vi "example.vi"() -> ()   [LabVIEW 2015]
doc: "Created by Artem Shevelev\nshevelev.pro\nartem@shevelev.pro\nLabVIEW Portal: https://labviewportal.org/memberlist.php?mode=viewprofile&u=2340"
uses:
  cluster_example_3.ctl
  cluster_example_1.ctl
  cluster_example_2.ctl
  ini_work_Library.lvlib
panel:
  out "data2":T1
  out "data1":T1
  out "default_values":bool
  out "error out":errorcluster
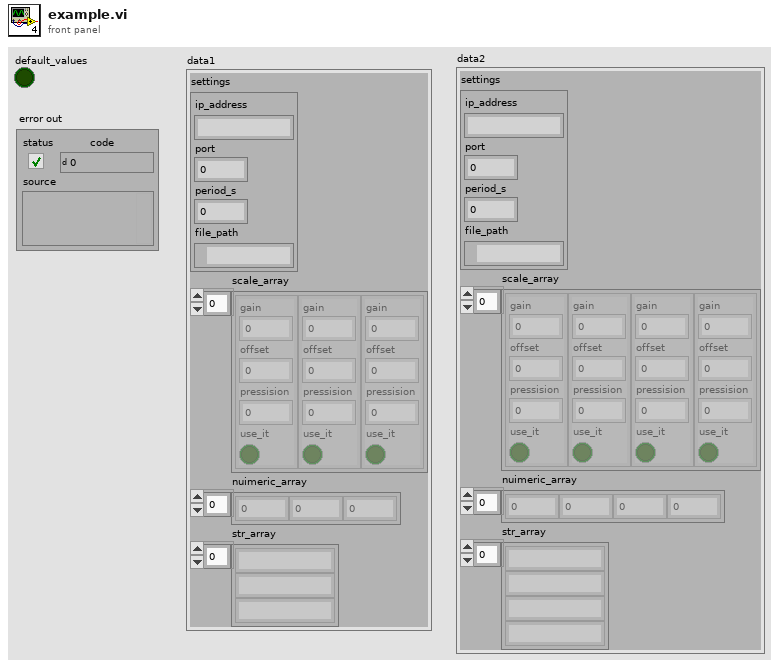
[diagram p1: front panel]
types:
  T1 = typedef "cluster_example_3.ctl" = cluster{"settings":T2, "scale_array":T3[], "nuimeric_array":dbl[], "str_array":string[]}
  T2 = typedef "cluster_example_1.ctl" = cluster{"ip_address":string, "port":i32, "period_s":dbl, "file_path":path}
  T3 = typedef "cluster_example_2.ctl" = cluster{"gain":dbl, "offset":dbl, "pressision":i32, "use_it":bool}
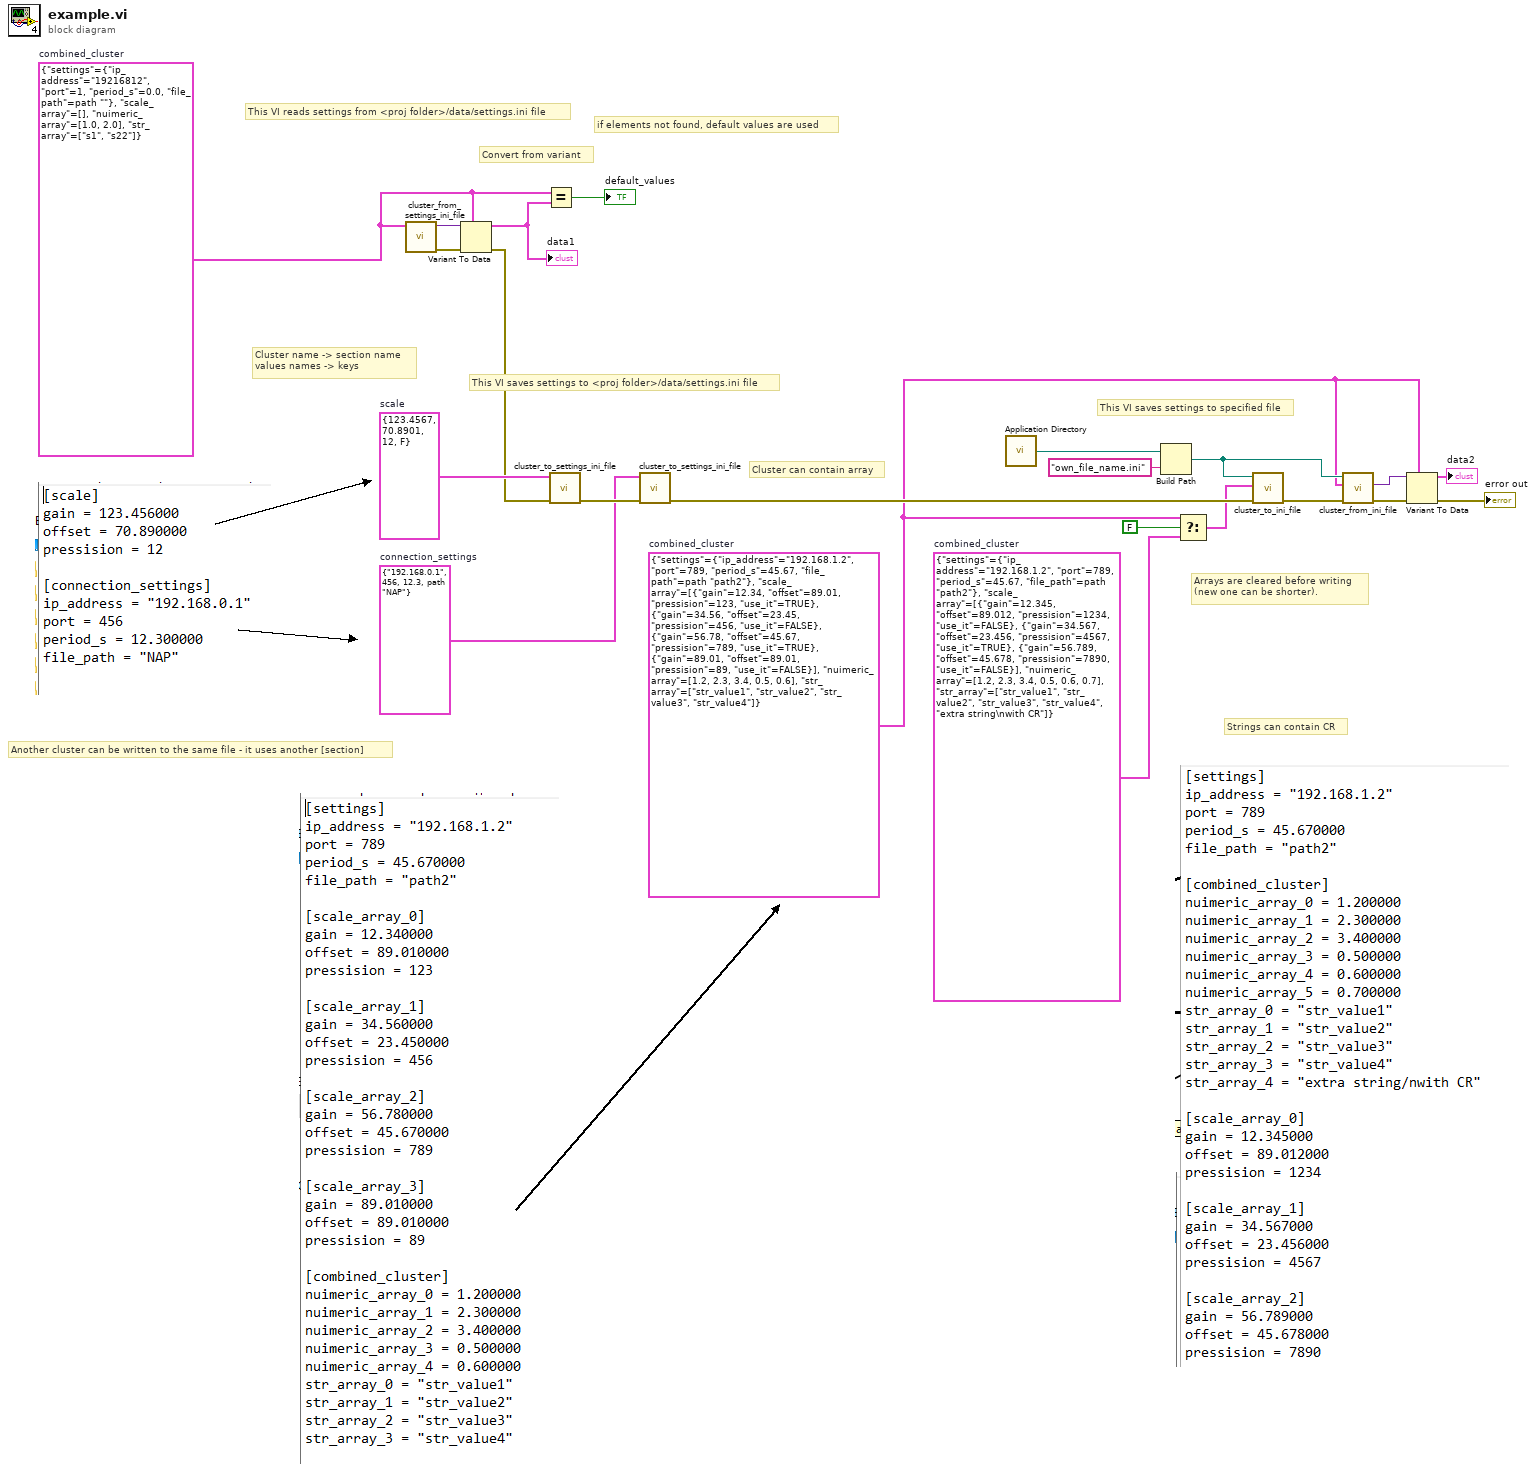
[diagram p0: block diagram]
diagram:
  w11 = T1 {"settings"={"ip_address"="19216812", "port"=1, "period_s"=0.0, "file_path"=path ""}, "scale_array"=[], "nuimeric_array"=[1.0, 2.0], "str_array"=["s1", "s22"]}  # combined_cluster
  w16 = T1 {"settings"={"ip_address"="192.168.1.2", "port"=789, "period_s"=45.67, "file_path"=path "path2"}, "scale_array"=[{"gain"=12.345, "offset"=89.012, "pressision"=1234, "use_it"=FALSE}, {"gain"=34.567, "offset"=23.456, "pressision"=4567, "use_it"=TRUE}, {"gain"=56.789, "offset"=45.678, "pressision"=7890, "use_it"=FALSE}], "nuimeric_array"=[1.2, 2.3, 3.4, 0.5, 0.6, 0.7], "str_array"=["str_value1", "str_value2", "str_value3", "str_value4", "extra string\nwith CR"]}  # combined_cluster
  w2 = T1 {"settings"={"ip_address"="192.168.1.2", "port"=789, "period_s"=45.67, "file_path"=path "path2"}, "scale_array"=[{"gain"=12.34, "offset"=89.01, "pressision"=123, "use_it"=TRUE}, {"gain"=34.56, "offset"=23.45, "pressision"=456, "use_it"=FALSE}, {"gain"=56.78, "offset"=45.67, "pressision"=789, "use_it"=TRUE}, {"gain"=89.01, "offset"=89.01, "pressision"=89, "use_it"=FALSE}], "nuimeric_array"=[1.2, 2.3, 3.4, 0.5, 0.6], "str_array"=["str_value1", "str_value2", "str_value3", "str_value4"]}  # combined_cluster
  w22 = T3 {"gain"=123.4567, "offset"=70.8901, "pressision"=12, "use_it"=FALSE}  # scale
  w20 = T2 {"ip_address"="192.168.0.1", "port"=456, "period_s"=12.3, "file_path"=path "NAP"}  # connection_settings
  # "if elements not found, default values are used"
  # "Convert from variant"
  # "This VI reads settings from <proj folder>/data/settings.ini file"
  # "Arrays are cleared before writing \n(new one can be shorter)."
  # "Strings can contain CR"
  # "Cluster can contain array"
  # "This VI saves settings to specified file"
  # "Another cluster can be written to the same file - it uses another [section]"
  # "Cluster name -> section name\nvalues names -> keys"
  # "This VI saves settings to <proj folder>/data/settings.ini file"
  n1 = call "cluster_from_settings_ini_file.vi"("containerIn"=w11) -> ("error out"=w12:errorcluster, "dataValue"=w13:variant)  [unwired: 9 in]
  n2 = Variant To Data(error in=w12, type=w11, Variant=w13) -> (data=w8:T1, error out=w9:errorcluster)
  "data1" <- w8
  n3 = Equal?(x=w11, y=w8) -> (x = y?=→"default_values":bool)
  n4 = call "cluster_to_settings_ini_file.vi"("error in (no error)"=w9, "containerIn"=w22) -> ("error out"=w21:errorcluster)  [unwired: 9 in]
  n5 = call "cluster_to_settings_ini_file.vi"("error in (no error)"=w21, "containerIn"=w20) -> ("error out"=w19:errorcluster)  [unwired: 9 in]
  n6 = call <vilib>:"Application Directory.vi"() -> ("Application Directory"=w17:path)
  n7 = Build Path(base path=w17, name or relative path="own_file_name.ini") -> (appended path=w5:path)
  n8 = Select(t=w2, s=FALSE, f=w16) -> (s? t:f=w15:T1)
  n9 = call "cluster_to_ini_file.vi"("error in (no error)"=w19, "data"=w15, "iniFilePath"=w5) -> ("error out"=w6:errorcluster)  [unwired: 8 in]
  n10 = call "cluster_from_ini_file.vi"("error in (no error)"=w6, "dataType"=w2, "iniFilePath"=w5) -> ("error out"=w4:errorcluster, "dataValue"=w3:variant)  [unwired: 7 in]
  n11 = Variant To Data(error in=w4, type=w2, Variant=w3) -> (data=→"data2":T1, error out=→"error out":errorcluster)
